vi "Process.vi"(8 "error in":errorcluster, 11 "SMO.Dictionary":refnum<class "SMO.Dictionary.lvclass">) -> (0 "error out":errorcluster, 3 "SMO.Dictionary out":refnum<class "SMO.Dictionary.lvclass">)   [LabVIEW 2013, in "SMO.Dictionary.lvlib" / "SMO.Dictionary.lvclass"]
doc: "---------------------------------------------------------------\nJKI State Machine Objects™\nhttp://jki.net/state-machine-objects/\nCopyright (C) 2005-2015, JKI <info@jki.net>\nALL RIGHTS RESERVED"
uses:
  SMO.Dictionary.lvclass
  <vilib>/JKI/JKI SMO/SMO/Typedefs/Parent Call--Enum.ctl
  <vilib>/JKI/JKI SMO/SMO/SMO.lvclass
  Typedefs/PrivateEvents--SMO.Dictionary.KeyValue-Pair.ctl
  Typedefs/PrivateEvents--SMO.Dictionary.GetMultipleValues.ctl
  Typedefs/PrivateEvents--SMO.Dictionary.KeyValue-Pair Array.ctl
  Typedefs/PrivateEvents--SMO.Dictionary.Get.ctl
  <vilib>/JKI/JKI SMO/SMO/SMO.lvclass/SMO.ctl
  <vilib>/JKI/JKI SMO/SMO/Private/ReftoDVR--SMO.vi
panel:
  # "For instructions on how to use the JKI State Machine Objects, examples and video tutorials, visit:\nhttp://jki.net/state-machine-objects/\n\nJKI State Machine Objects™\nhttp://jki.net/state-machine-objects/\nCopyright (C) 2005-2015, JKI <info@jki.net>\nALL RIGHTS RESERVED"
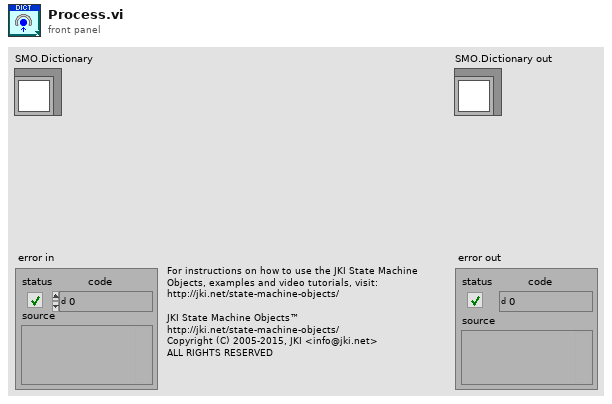
[diagram p1: front panel]
types:
  T1 = typedef "SMO.lvclass/Parent Call--Enum.ctl" = enum16{"Allows parent to run", "Does not request parent to run"}
  T2 = enum32{"invalid app kind", "Development System", "Run Time System", "Student Edition", "Embedded LabVIEW", "Evaluation", "Custom"}
  T3 = enum32{"Invalid", "Standard", "Closed", "Hidden", "Minimized", "Maximized"}
  T4 = enum32{"Bad", "Idle", "Run top level", "Running"}
  T5 = typedef "SMO.Dictionary.lvlib/SMO.Dictionary.lvclass/PrivateEvents--SMO.Dictionary.KeyValue-Pair.ctl" = cluster{"Key":string, "Value":variant}
  T6 = typedef "SMO.Dictionary.lvlib/SMO.Dictionary.lvclass/PrivateEvents--SMO.Dictionary.KeyValue-Pair Array.ctl" = cluster{"Keys":string[], "Values":variant[]}
  T7 = typedef "SMO.Dictionary.lvlib/SMO.Dictionary.lvclass/PrivateEvents--SMO.Dictionary.Get.ctl" = cluster{"Key":string, "response":refnum<notifier>}
  T8 = typedef "SMO.Dictionary.lvlib/SMO.Dictionary.lvclass/PrivateEvents--SMO.Dictionary.GetMultipleValues.ctl" = cluster{"Keys":string[], "response":refnum<notifier>}
  T9 = cluster{"Core":cluster{"Current VI Reference":refnum<vi>, "Close Panel on Exit?":bool, "error":errorcluster}, "Self Reference":refnum<class "SMO.Dictionary.lvclass">, "KeyValue Pair":T5, "Get":T7, "GetMultiple":T8}
  T10 = cluster{"Current VI Reference":refnum<vi>, "Close Panel on Exit?":bool, "error":errorcluster}
  T11 = typedef "SMO.lvclass/Protected Events.ctl" = cluster{"StopProcesses":refnum<user-event>, "AbortProcesses":refnum<user-event>, "Config Changed":refnum<user-event>, "Dependency":refnum<user-event>}
  T12 = typedef "SMO.Dictionary.lvlib/SMO.Dictionary.lvclass/PrivateEvents--Cluster.ctl" = cluster{"Update":refnum<user-event>, "Clear Dictionary":refnum<user-event>, "Delete":refnum<user-event>, "Get":refnum<user-event>, "GetMultiple":refnum<user-event>}
  T13 = typedef "SMO.Dictionary.lvlib/SMO.Dictionary.lvclass/PublicEvents--Cluster.ctl" = cluster{"Cleared":refnum<user-event>, "Deleted":refnum<user-event>, "Updated":refnum<user-event>}
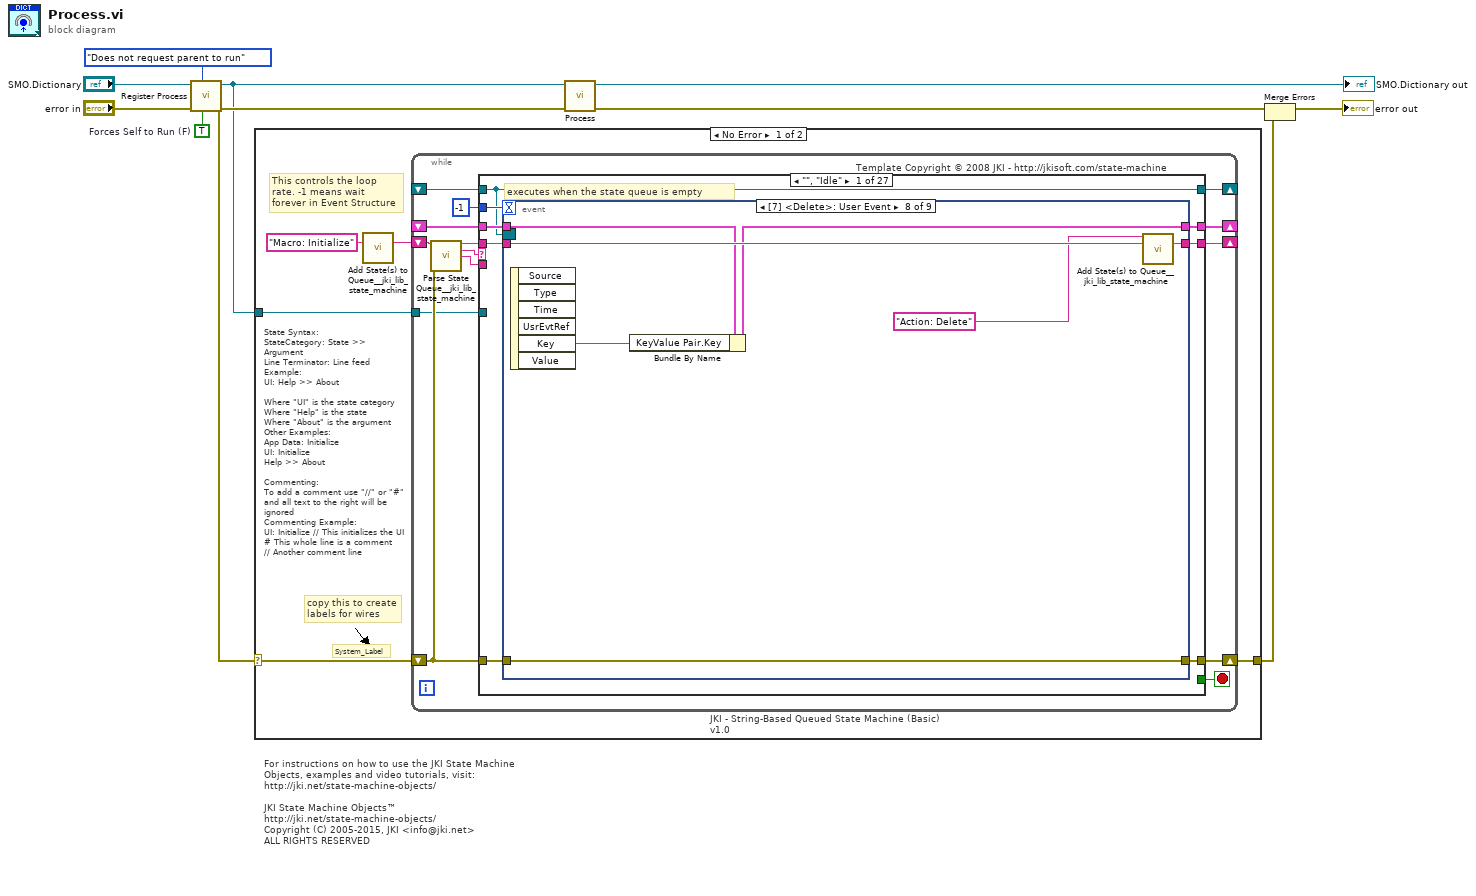
[diagram p0: block diagram]
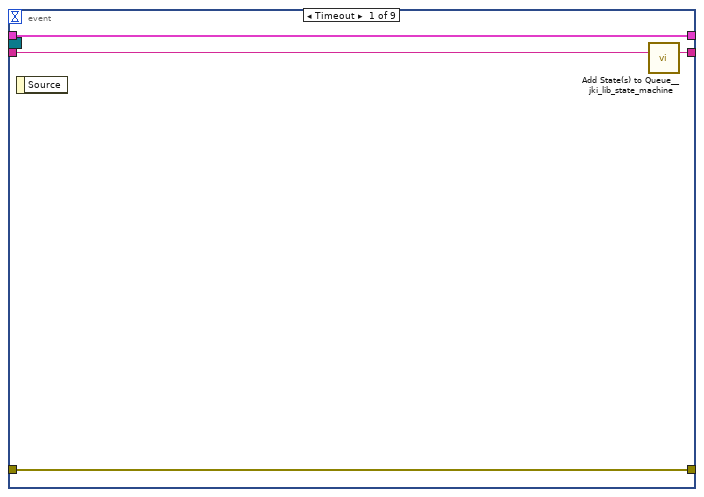
[diagram p2: hidden frame]
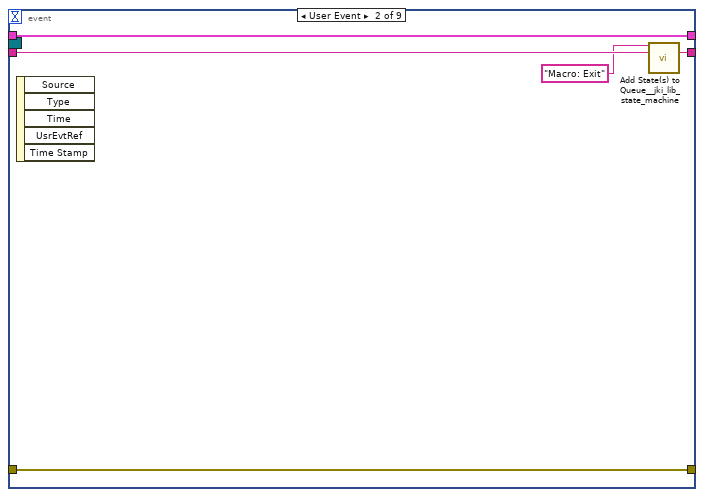
[diagram p3: hidden frame]
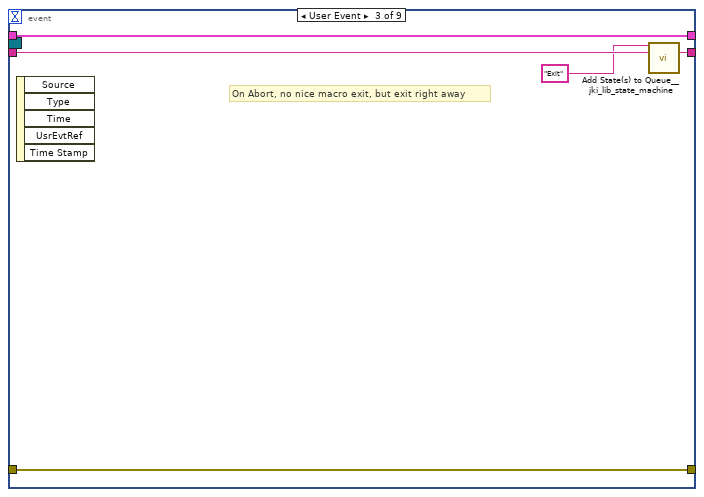
[diagram p4: hidden frame]
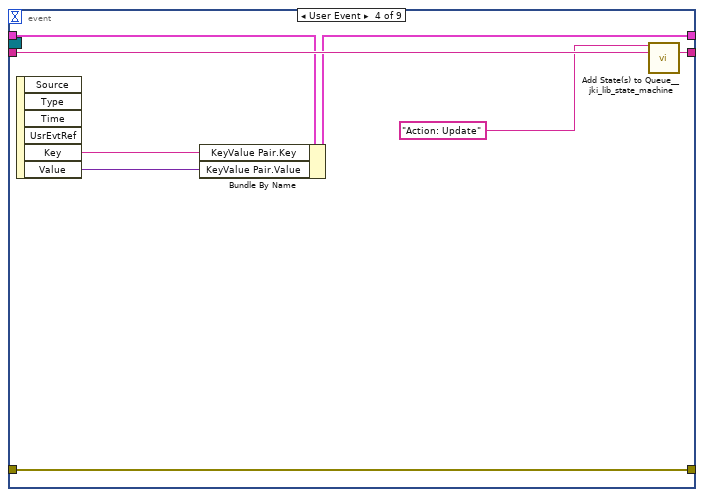
[diagram p5: hidden frame]
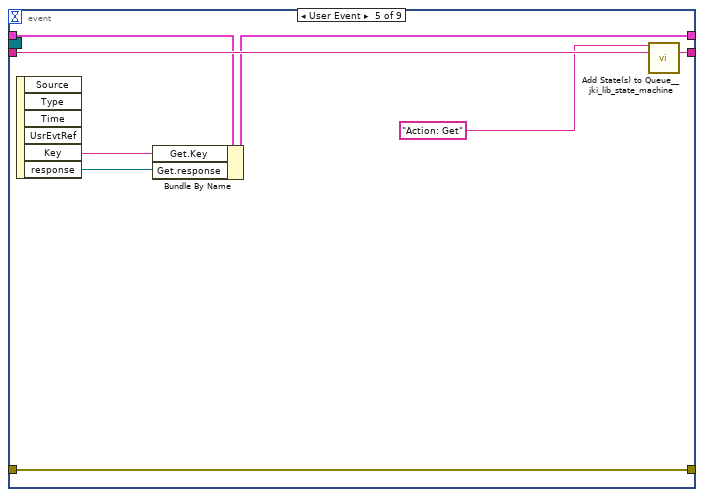
[diagram p6: hidden frame]
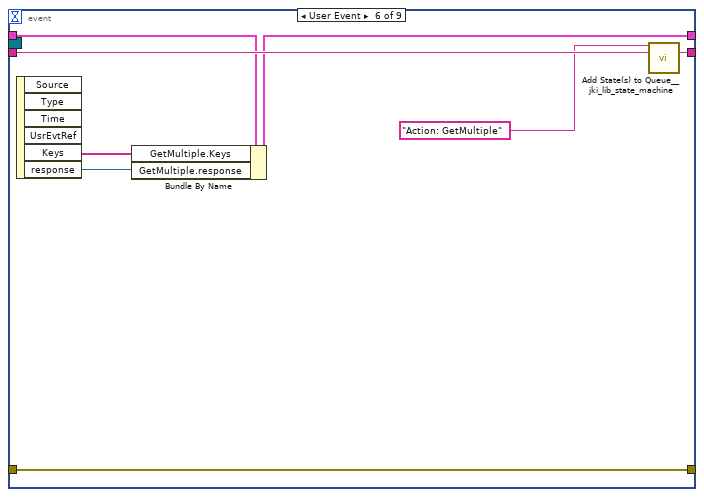
[diagram p7: hidden frame]
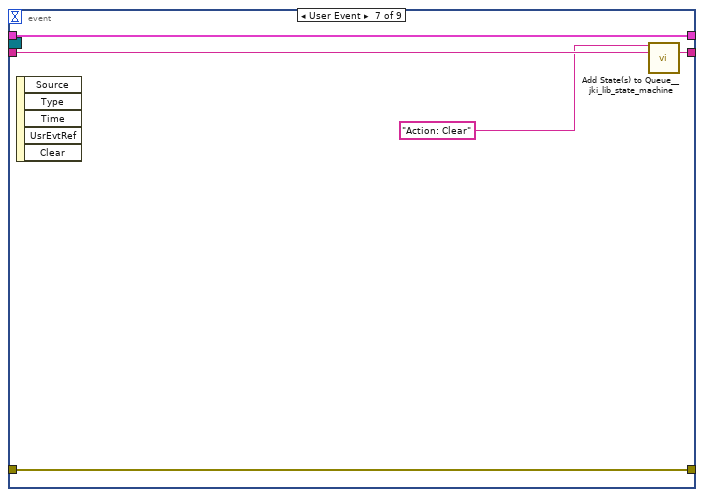
[diagram p8: hidden frame]
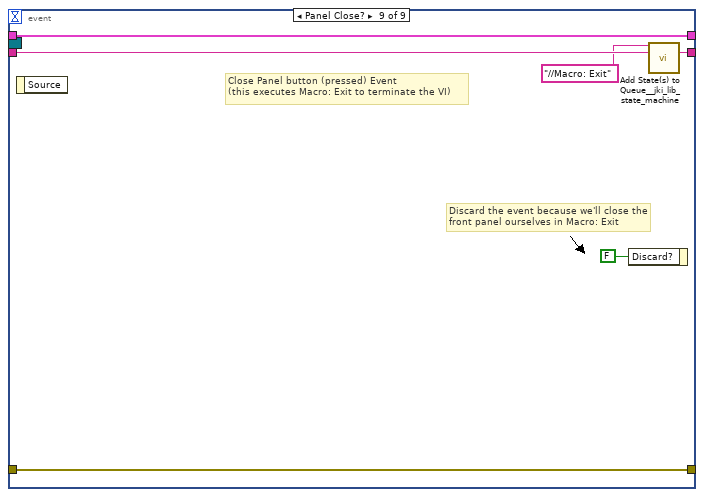
[diagram p9: hidden frame]
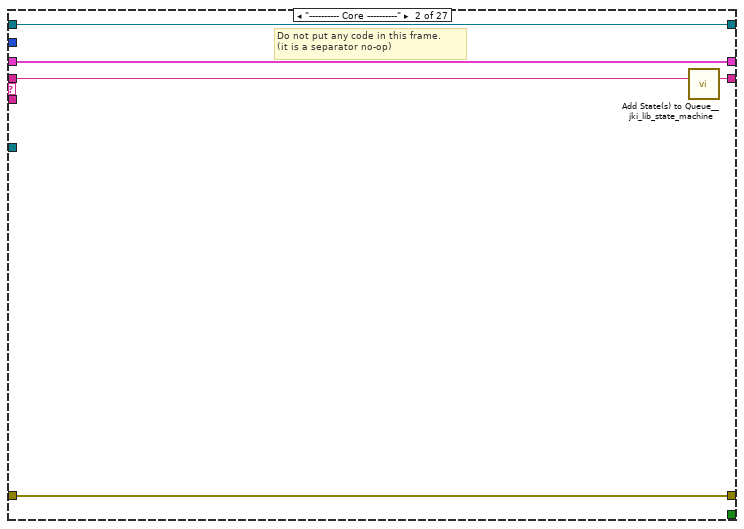
[diagram p10: hidden frame]
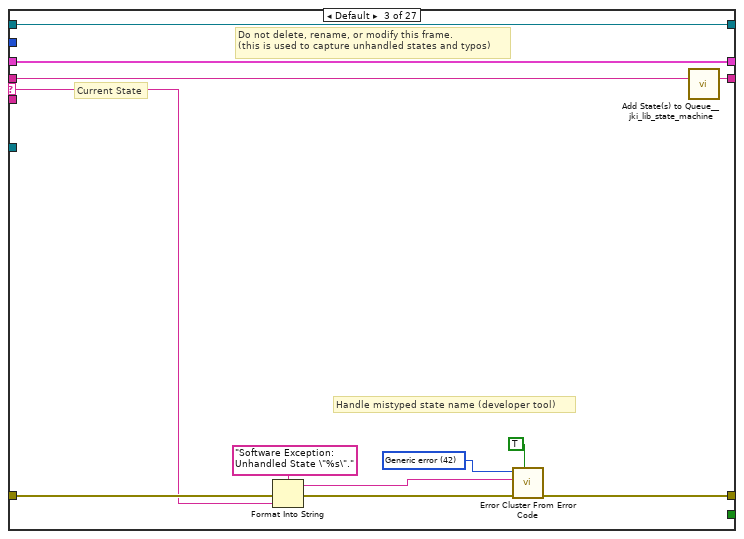
[diagram p11: hidden frame]
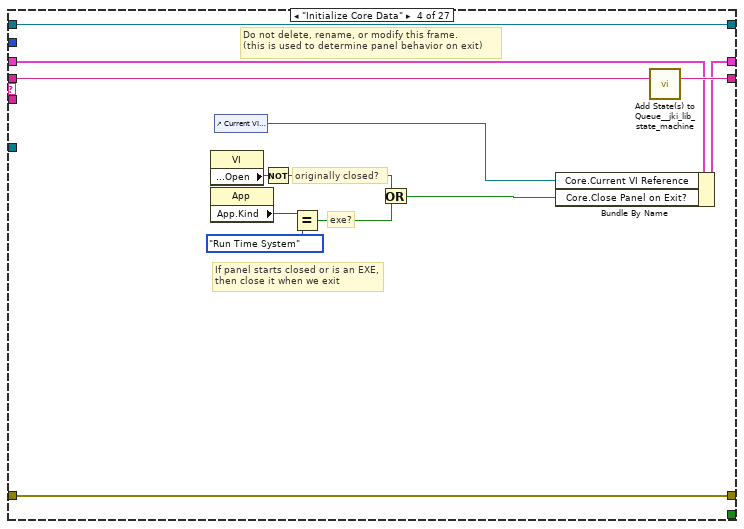
[diagram p12: hidden frame]
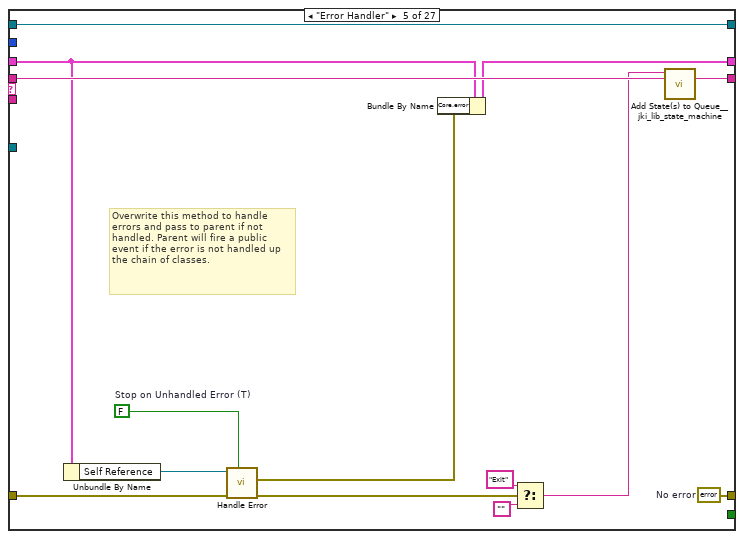
[diagram p13: hidden frame]
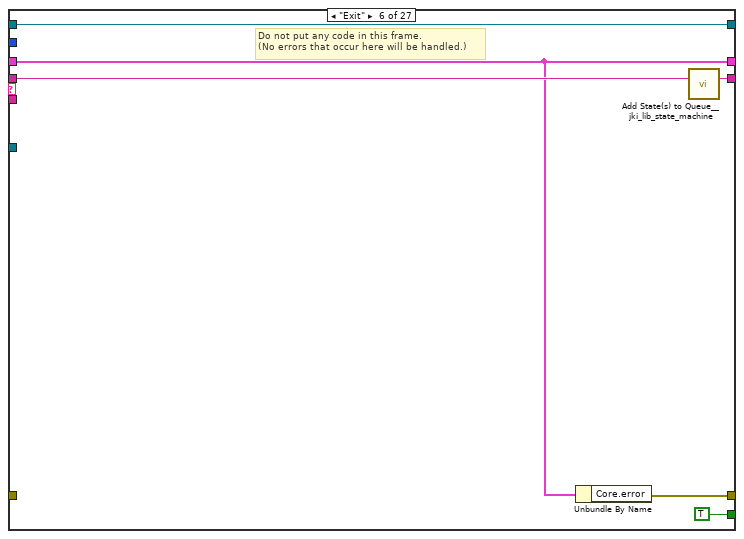
[diagram p14: hidden frame]
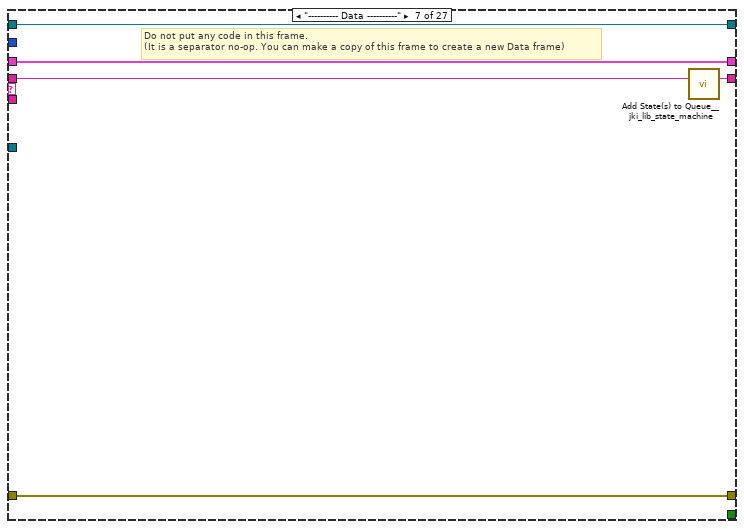
[diagram p15: hidden frame]
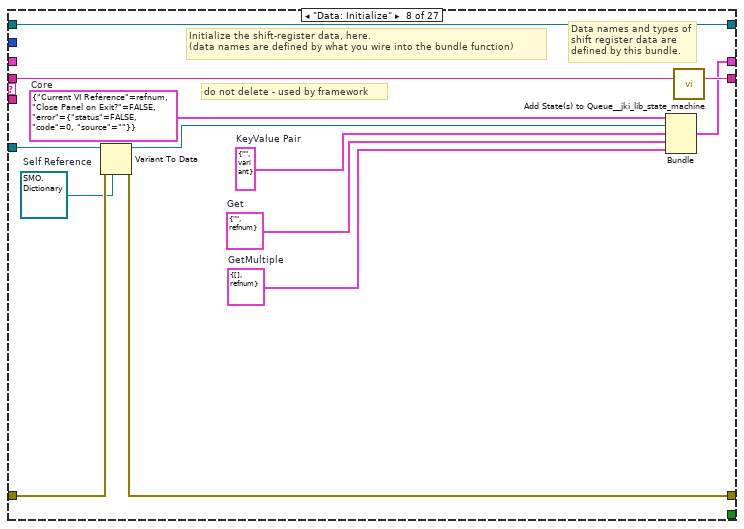
[diagram p16: hidden frame]
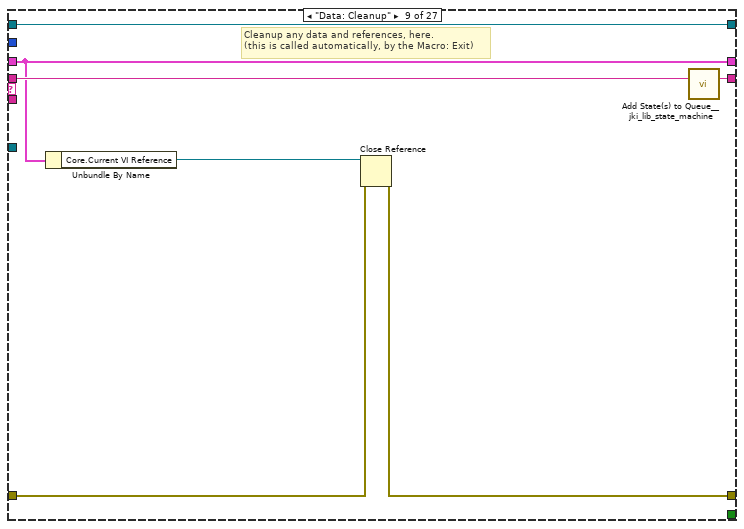
[diagram p17: hidden frame]
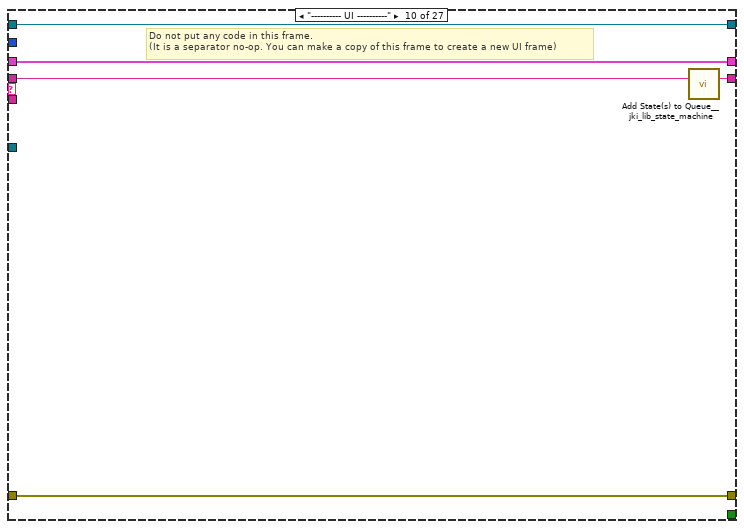
[diagram p18: hidden frame]
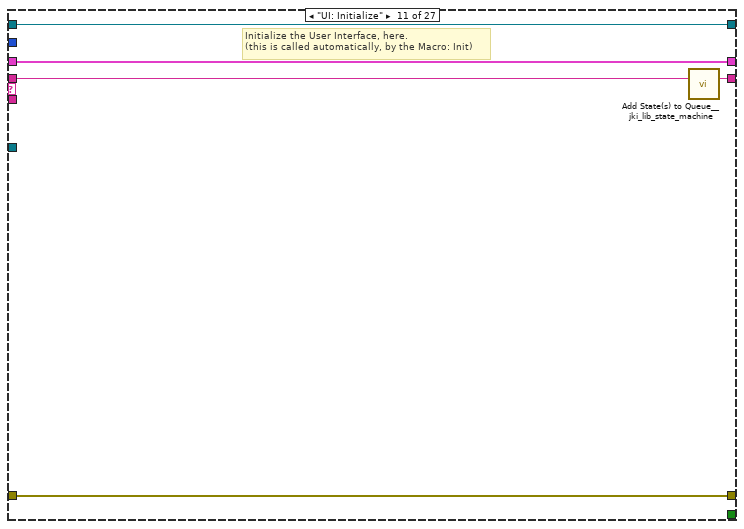
[diagram p19: hidden frame]
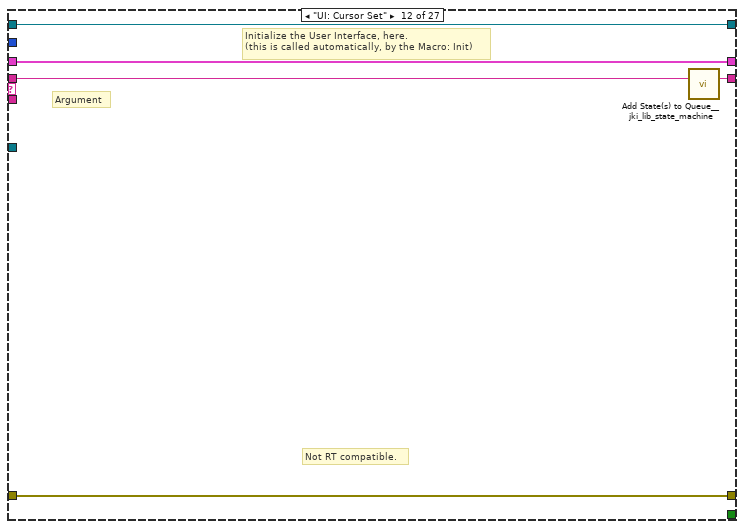
[diagram p20: hidden frame]
diagram:
  w1 = TRUE  # Forces Self to Run (F)
  # "For instructions on how to use the JKI State Machine Objects, examples and video tutorials, visit:\nhttp://jki.net/state-machine-objects/\n\nJKI State Machine Objects™\nhttp://jki.net/state-machine-objects/\nCopyright (C) 2005-2015, JKI <info@jki.net>\nALL RIGHTS RESERVED"
  n1 = call <vilib>:"Register Process.vi"("Forces Self to Run (F)"=w1, "Parent Call"=Parent_Call--Enum."Does not request parent to run", "error in (no error)"="error in", "SMO"="SMO.Dictionary") -> ("error out"=w7:errorcluster, "SMO out"=w6:refnum<class "SMO.Dictionary.lvclass">)  [unwired: 6 in]
  n2 = case shown="No Error" w7 {
    selector: w7 -> [w12 w372]
    tunnel: w6 -> [w13 _]
    tunnel: [w11 w372] -> w3
    frame No Error {
      # "State Syntax:\nStateCategory: State >> Argument\nLine Terminator: Line feed\nExample:\nUI: Help >> About\n\nWhere \"UI\" is the state category\nWhere \"Help\" is the state\nWhere \"About\" is the argument\nOther Examples:\nApp Data: Initialize\nUI: Initialize\nHelp >> About\n\nCommenting:\nTo add a comment use \"//\" or \"#\" and all text to the right will be ignored\nCommenting Example:\nUI: Initialize // This initializes the UI\n# This whole line is a comment\n// Another comment line"
      # "copy this to create labels for wires"
      # "This controls the loop rate. -1 means wait forever in Event Structure"
      # "System_Label"
      n3 = call <vilib>:"Add State(s) to Queue__jki_lib_state_machine.vi"("State(s) in (\"\")"="Macro: Initialize") -> ("States Out"=w15:string)  [unwired: 14 in]
      n4 = while "JKI - String-Based Queued State Machine (Basic) v1.0" {
        shift-right: [w22] -> _
        shift-left: _ -> [w21]
        shift-right: [w25] -> w11
        shift-left: w12 -> [w19]
        shift-right: [w24] -> _
        shift-left: w15 -> [w26]
        tunnel: w13 -> [w18]
        shift-right: [w17] -> _
        shift-left: _ -> [w16]
        stop <- w23 stop-if-true
        # "Template Copyright © 2008 JKI - http://jkisoft.com/state-machine"
        n5 = call <vilib>:"Parse State Queue__jki_lib_state_machine.vi"("State Queue"=w26, "Error In (no error)"=w19) -> ("Remaining States"=w28:string, "Current State"=w29:string, "Arguments"=w27:string)  [unwired: 11 in]
        n6 = case shown="\"\", \"Idle\"" w29 {
          selector: w29 -> [_ _ w100 _ _ _ _ _ _ _ _ _ _ _ _ _ _ _ _ _ _ _ _ _ _ _ _]
          tunnel: w28 -> [w37 w98 w104 w123 w137 w143 w148 w161 w168 w173 w178 w183 w191 w223 w237 w251 w256 w267 w272 w292 w298 w303 w314 w330 w346 w356 w371]
          tunnel: w27 -> [_ _ _ _ _ _ _ _ _ _ _ _ w185 _ _ _ _ _ _ _ _ _ _ _ _ _ _]
          tunnel: w21 -> [w35 w95 w102 w114 w131 w139 w145 _ w163 w170 w176 w181 w187 w220 w233 w242 w253 w264 w269 w290 w296 w301 w311 w327 w343 w353 w368]
          tunnel: [w34 w96 w106 w120 w132 w138 w146 w157 w164 w171 w175 w179 w188 w221 w235 w249 w254 w258 w270 w283 w294 w299 w304 w317 w341 w347 w358] -> w25
          tunnel: w19 -> [w33 w96 w105 w120 w133 _ w146 w158 w165 w171 w175 w179 w189 w221 w235 w249 w254 w259 w270 w287 w294 w299 w308 w315 w333 w349 w365]
          tunnel: [w36 w97 w103 w122 w136 w142 w147 w160 w167 w172 w177 w182 w190 w222 w236 w250 w255 w266 w271 w291 w297 w302 w313 w329 w345 w355 w370] -> w24
          tunnel: [_ _ _ _ _ TRUE _ _ _ _ _ _ _ _ _ _ _ _ _ _ _ _ _ _ _ _ _] -> w23
          tunnel: [w32 w95 w102 w121 w130 w139 w145 w159 w163 w170 w176 w181 w187 w220 w233 w242 w253 w264 w269 w290 w296 w301 w310 w326 w342 w352 w367] -> w22
          tunnel: -1 ("Timeout") -> [w31 _ _ _ _ _ _ _ _ _ _ _ _ _ _ _ _ _ _ _ _ _ _ _ _ _ _]
          tunnel: w18 -> [_ _ _ _ _ _ _ w155 _ _ _ _ _ _ _ _ _ _ _ _ _ _ _ _ _ _ _]
          tunnel: [w30 w94 w99 w111 w135 w140 w144 w153 w162 w169 w174 w180 w184 w219 w234 w243 w252 w265 w268 w273 w295 w300 w312 w328 w344 w354 w369] -> w17
          tunnel: w16 -> [w30 w94 w99 w111 w135 w140 w144 w153 w162 w169 w174 w180 w184 w219 w234 w243 w252 w265 w268 _ w295 w300 w312 w328 w344 w354 w369]
          frame "", "Idle" {
            # "executes when the state queue is empty"
            n7 = event shown="[7] <Delete>: User Event" {
              selector: w30 -> [_ _ _ _ _ _ _ _ _]
              dyn-events: _ -> [_ _ _ _ _ _ _ _ _]
              timeout: w31 -> [_ _ _ _ _ _ _ _ _]
              tunnel: w37 -> [w41 w46 w51 w59 w67 w75 w80 w87 w93]
              tunnel: [w40 w45 w50 w58 w66 w74 w79 w86 w92] -> w36
              tunnel: w35 -> [w39 w43 w48 w54 w62 w71 w76 w82 w90]
              tunnel: [w38 w44 w49 w57 w65 w73 w78 w85 w91] -> w34
              tunnel: w33 -> [w38 w44 w49 w57 w65 w73 w78 w85 w91]
              tunnel: [w39 w43 w48 w53 w61 w70 w76 w81 w90] -> w32
              event Timeout {
                n8 = event-data() -> ()  [unwired: 1 in, 1 out]
                n9 = call <vilib>:"Add State(s) to Queue__jki_lib_state_machine.vi"("State(s) in (\"\")"=w41) -> ("States Out"=w40:string)  [unwired: 14 in]
              }
              event User Event {
                n10 = event-data() -> ()  [unwired: 1 in, 5 out]
                n11 = call <vilib>:"Add State(s) to Queue__jki_lib_state_machine.vi"("State(s) in Front (\"\")"="Macro: Exit", "State(s) in (\"\")"=w46) -> ("States Out"=w45:string)  [unwired: 13 in]
              }
              event User Event {
                # "On Abort, no nice macro exit, but exit right away"
                n12 = event-data() -> ()  [unwired: 1 in, 5 out]
                n13 = call <vilib>:"Add State(s) to Queue__jki_lib_state_machine.vi"("State(s) in Front (\"\")"="Exit", "State(s) in (\"\")"=w51) -> ("States Out"=w50:string)  [unwired: 13 in]
              }
              event User Event {
                n14 = event-data() -> ("Key"=w56:string, "Value"=w55:variant)  [unwired: 1 in, 4 out]
                n15 = Bundle By Name(cluster=w54, "KeyValue Pair.Key"=w56, "KeyValue Pair.Value"=w55) -> (w53:T9)
                n16 = call <vilib>:"Add State(s) to Queue__jki_lib_state_machine.vi"("State(s) in Front (\"\")"="Action: Update", "State(s) in (\"\")"=w59) -> ("States Out"=w58:string)  [unwired: 13 in]
              }
              event User Event {
                n17 = event-data() -> ("Key"=w64:string, "response"=w63:refnum<notifier>)  [unwired: 1 in, 4 out]
                n18 = Bundle By Name(cluster=w62, "Get.Key"=w64, "Get.response"=w63) -> (w61:T9)
                n19 = call <vilib>:"Add State(s) to Queue__jki_lib_state_machine.vi"("State(s) in Front (\"\")"="Action: Get", "State(s) in (\"\")"=w67) -> ("States Out"=w66:string)  [unwired: 13 in]
              }
              event User Event {
                n20 = event-data() -> ("Keys"=w72:string[], "response"=w68:refnum<notifier>)  [unwired: 1 in, 4 out]
                n21 = Bundle By Name(cluster=w71, "GetMultiple.Keys"=w72, "GetMultiple.response"=w68) -> (w70:T9)
                n22 = call <vilib>:"Add State(s) to Queue__jki_lib_state_machine.vi"("State(s) in Front (\"\")"="Action: GetMultiple", "State(s) in (\"\")"=w75) -> ("States Out"=w74:string)  [unwired: 13 in]
              }
              event User Event {
                n23 = event-data() -> ()  [unwired: 1 in, 5 out]
                n24 = call <vilib>:"Add State(s) to Queue__jki_lib_state_machine.vi"("State(s) in Front (\"\")"="Action: Clear", "State(s) in (\"\")"=w80) -> ("States Out"=w79:string)  [unwired: 13 in]
              }
              event User Event {
                n25 = event-data() -> ("Key"=w83:string)  [unwired: 1 in, 5 out]
                n26 = Bundle By Name(cluster=w82, "KeyValue Pair.Key"=w83) -> (w81:T9)
                n27 = call <vilib>:"Add State(s) to Queue__jki_lib_state_machine.vi"("State(s) in Front (\"\")"="Action: Delete", "State(s) in (\"\")"=w87) -> ("States Out"=w86:string)  [unwired: 13 in]
              }
              event Panel Close? {
                # "Discard the event because we'll close the front panel ourselves in Macro: Exit"
                # "Close Panel button (pressed) Event\n(this executes Macro: Exit to terminate the VI)"
                n28 = event-data() -> ()  [unwired: 1 in, 1 out]
                n29 = event-data("Discard?"=FALSE) -> ()  [unwired: 1 in, 1 out]
                n30 = call <vilib>:"Add State(s) to Queue__jki_lib_state_machine.vi"("State(s) in Front (\"\")"="//Macro: Exit", "State(s) in (\"\")"=w93) -> ("States Out"=w92:string)  [unwired: 13 in]
              }
            }
          }
          frame "---------- Core ----------" {
            # "Do not put any code in this frame.\n(it is a separator no-op)"
            n31 = call <vilib>:"Add State(s) to Queue__jki_lib_state_machine.vi"("State(s) in (\"\")"=w98) -> ("States Out"=w97:string)  [unwired: 14 in]
          }
          frame Default {
            w109 = 42 items=["No error", "Argument error", "Memory is full", "Out of zone", "End of file", "File already open", "Generic file I/O error", "File not found", "File permission error", "Disk is full", "Duplicate path", "Too many files open", "System feature not enabled", "Resource file not found", "Cannot add resource", "Resource not found", "Image not found", "Image memory error", "Pen does not exist", "Config type invalid", "Config token not found", "Config parse error", "Config memory error", "Bad external code format", "Bad external code offset", "External code not present", "Null window", "Destroy window error", "Null menu", "Print aborted", "Bad print record", "Print driver error", "Windows error during printing", "Memory error during printing", "Print dialog error", "Generic print error", "Invalid device refnum", "Device not found", "Device parameter error", "Device unit error", "Cannot open device", "Device call aborted", "Generic error", "Cancelled by user", "Object ID too low", "Object ID too high", "Object not in heap", "Unknown heap", "Unknown object (invalid DefProc)", "Unknown object (DefProc not in table)", "Message out of range", "Invalid (null) method", "Unknown message", "Manager call not supported", "Bad address", "Network operation in progress", "Network operation timed out", "Connection is busy", "Network attribute not supported", "Network error", "Address in use", "System out of memory", "Connection aborted", "Connection refused", "Not connected", "Already connected", "Connection closed", "Initialization error (interapplication manager)", "Bad occurrence", "Wait on unbound occurrence handler", "Occurrence queue overflow", "Datalog type conflict", "Unused", "Unrecognized type (interapplication manager)", "Memory corrupt", "Failed to make temporary DLL", "Old CIN version", "Drag socket not found", "Failed to load drop-object", "Failed to register OLE object", "Failed to release OLE object", "Format specifier type mismatch", "Unknown format specifier", "Too few format specifiers", "Too many format specifiers", "Scan failed", "Newer CIN version", "Error converting to variant", "Runtime menu error", "Password tampered", "Variant attribute not found", "Incompatible variant data type", "Event data is not available", "Event Store is not present", "Occurrence is not found", "Event Queue is not created", "Event info is not available", "Refnum passed is NULL", "Error retrieving Class GUID", "Error retrieving CoClass GUID", "Error retrieving TypeLib GUID.", "Bad built application magic bytes.", "Specific driver is different from the specific driver associated with the Logical Name.", "There is no session opened to the class driver.", "Max Error", "MAX - Error with config objects", "MAX - Error loading configuration", "MAX - Group not supported"]
            # "Current State"
            # "Do not delete, rename, or modify this frame.\n(this is used to capture unhandled states and typos)"
            # "Handle mistyped state name (developer tool)"
            n32 = Format Into String(format string="Software Exception: Unhandled State \"%s\"." ("message"), error in=w105, w100) -> (resulting string=w108:string, error out=w107:errorcluster)  [unwired: 1 in]
            n33 = call <vilib>:"Error Cluster From Error Code.vi"("show call chain? (False)"=TRUE, "error in (no error)"=w107, "error message (\"\")"=w108, "error code (0)"=w109) -> ("error out"=w106:errorcluster)  [unwired: 5 in]
            n34 = call <vilib>:"Add State(s) to Queue__jki_lib_state_machine.vi"("State(s) in (\"\")"=w104) -> ("States Out"=w103:string)  [unwired: 14 in]
          }
          frame "Initialize Core Data" {
            # "Do not delete, rename, or modify this frame.\n(this is used to determine panel behavior on exit)"
            # "originally closed?"
            # "exe?"
            # "If panel starts closed or is an EXE, then close it when we exit"
            n35 = property class="VI"() -> ("Front Panel.Open"=w119:bool)  [unwired: 2 in, 2 out]
            n36 = property class="App"() -> ("App.Kind"=w118:T2)  [unwired: 2 in, 2 out]
            n37 = control-ref of="Current VI Reference"() -> (w112:refnum<vi>)
            n38 = Not(x=w119) -> (.not. x?=w116:bool)
            n39 = Equal?(x=w118, y=T2."Run Time System" ("Application:Kind")) -> (x = y?=w115:bool)
            n40 = Or(x=w116, y=w115) -> (x .or. y?=w113:bool)
            n41 = Bundle By Name(cluster=w114, "Core.Current VI Reference"=w112, "Core.Close Panel on Exit?"=w113) -> (w121:T9)
            n42 = call <vilib>:"Add State(s) to Queue__jki_lib_state_machine.vi"("State(s) in (\"\")"=w123) -> ("States Out"=w122:string)  [unwired: 14 in]
          }
          frame "Error Handler" {
            w124 = FALSE  # Stop on Unhandled Error (T)
            w132 = errorcluster {"status"=FALSE, "code"=0, "source"=""}  # No error
            # "Overwrite this method to handle errors and pass to parent if not handled. Parent will fire a public event if the error is not handled up the chain of classes."
            n43 = Unbundle By Name(w131) -> ("Self Reference"=w134:refnum<class "SMO.Dictionary.lvclass">)
            n44 = call-dynamic "Handle Error.vi"("Stop on Unhandled Error (T)"=w124, "error in"=w133, "SMO.Dictionary"=w134) -> ("handling error"=w125:errorcluster, "Unhandled error"=w128:errorcluster)  [unwired: 6 in, 1 out]
            n45 = Bundle By Name(cluster=w131, "Core.error"=w128) -> (w130:T9)
            n46 = Select(t="Exit", s=w125, f="") -> (s? t:f=w129:string)
            n47 = call <vilib>:"Add State(s) to Queue__jki_lib_state_machine.vi"("State(s) in Front (\"\")"=w129, "State(s) in (\"\")"=w137) -> ("States Out"=w136:string)  [unwired: 13 in]
          }
          frame "Exit" {
            # "Do not put any code in this frame.\n(No errors that occur here will be handled.)"
            n48 = Unbundle By Name(w139) -> ("Core.error"=w138:errorcluster)
            n49 = call <vilib>:"Add State(s) to Queue__jki_lib_state_machine.vi"("State(s) in (\"\")"=w143) -> ("States Out"=w142:string)  [unwired: 14 in]
          }
          frame "---------- Data ----------" {
            # "Do not put any code in this frame.\n(It is a separator no-op. You can make a copy of this frame to create a new Data frame)"
            n50 = call <vilib>:"Add State(s) to Queue__jki_lib_state_machine.vi"("State(s) in (\"\")"=w148) -> ("States Out"=w147:string)  [unwired: 14 in]
          }
          frame "Data: Initialize" {
            w149 = T7 {"Key"="", "response"=refnum}  # Get
            w150 = T8 {"Keys"=[], "response"=refnum}  # GetMultiple
            w151 = T5 {"Key"="", "Value"=variant}  # KeyValue Pair
            w152 = T10 {"Current VI Reference"=refnum, "Close Panel on Exit?"=FALSE, "error"={"status"=FALSE, "code"=0, "source"=""}}  # Core
            w156 = refnum<class "SMO.Dictionary.lvclass"> refnum  # Self Reference
            # "do not delete - used by framework"
            # "Data names and types of shift register data are defined by this bundle."
            # "Initialize the shift-register data, here.\n(data names are defined by what you wire into the bundle function)"
            n51 = Variant To Data(error in=w158, type=w156, Variant=w155) -> (data=w154:refnum<class "SMO.Dictionary.lvclass">, error out=w157:errorcluster)
            n52 = Bundle("Core"=w152, "Self Reference"=w154, "KeyValue Pair"=w151, "Get"=w149, "GetMultiple"=w150) -> (w159:T9)  [unwired: 1 in]
            n53 = call <vilib>:"Add State(s) to Queue__jki_lib_state_machine.vi"("State(s) in (\"\")"=w161) -> ("States Out"=w160:string)  [unwired: 14 in]
          }
          frame "Data: Cleanup" {
            # "Cleanup any data and references, here.\n(this is called automatically, by the Macro: Exit)"
            n54 = Unbundle By Name(w163) -> ("Core.Current VI Reference"=w166:refnum<vi>)
            n55 = Close Reference(reference=w166, error in (no error)=w165) -> (error out=w164:errorcluster)
            n56 = call <vilib>:"Add State(s) to Queue__jki_lib_state_machine.vi"("State(s) in (\"\")"=w168) -> ("States Out"=w167:string)  [unwired: 14 in]
          }
          frame "---------- UI ----------" {
            # "Do not put any code in this frame.\n(It is a separator no-op. You can make a copy of this frame to create a new UI frame)"
            n57 = call <vilib>:"Add State(s) to Queue__jki_lib_state_machine.vi"("State(s) in (\"\")"=w173) -> ("States Out"=w172:string)  [unwired: 14 in]
          }
          frame "UI: Initialize" {
            # "Initialize the User Interface, here.\n(this is called automatically, by the Macro: Init)"
            n58 = call <vilib>:"Add State(s) to Queue__jki_lib_state_machine.vi"("State(s) in (\"\")"=w178) -> ("States Out"=w177:string)  [unwired: 14 in]
          }
          frame "UI: Cursor Set" {
            # "Not RT compatible."
            # "Argument"
            # "Initialize the User Interface, here.\n(this is called automatically, by the Macro: Init)"
            n59 = call <vilib>:"Add State(s) to Queue__jki_lib_state_machine.vi"("State(s) in (\"\")"=w183) -> ("States Out"=w182:string)  [unwired: 14 in]
          }
          frame "UI: Front Panel State" {
            # "Argument"
            # "Set Front Panel Open or Closed\n(Usage: \"UI: Front Panel State >> Open|Close\")"
            n60 = Unbundle By Name(w187) -> ("Core.Current VI Reference"=w186:refnum<vi>)
            n61 = disable-structure shown="Default" {
              disable-tunnel: w189 -> [w195 w218]
              disable-tunnel: [w194 w218] -> w188
              disable-tunnel: w186 -> [w193 _]
              disable-tunnel: w185 -> [w192 _]
              frame condition #0 (active) {
                n62 = case shown="\"Close\"" w192 {
                  tunnel: w195 -> [w199 w212]
                  tunnel: [w201 w213] -> w194
                  tunnel: w193 -> [w200 w210]
                  frame "Open", Default {
                    n63 = property class="VI"(reference=w200, error in=w199) -> (reference out=w197:refnum<vi>, error out=w198:errorcluster, "FP.State"=w196:T3)
                    n64 = case shown="\"Closed\"" w196 {
                      tunnel: [w204 w207] -> w201
                      tunnel: w198 -> [w203 w207]
                      tunnel: w197 -> [w202 _]
                      frame "Closed" {
                        n65 = invoke class="VI" method="FP.Open"(reference=w202, error in=w203, "Activate"=TRUE, "State"=T3."Standard") -> (error out=w204:errorcluster)  [unwired: 1 in, 4 out]
                      }
                      frame Default {
                      }
                    }
                  }
                  frame "Close" {
                    n66 = property class="VI"(reference=w210, error in=w212) -> (reference out=w209:refnum<vi>, error out=w211:errorcluster, "FP.State"=w208:T3)
                    n67 = case shown="Default" w208 {
                      tunnel: [w214 w217] -> w213
                      tunnel: w211 -> [w214 w216]
                      tunnel: w209 -> [_ w215]
                      frame "Invalid", "Closed" {
                      }
                      frame Default {
                        n68 = invoke class="VI" method="FP.Close"(reference=w215, error in=w216) -> (error out=w217:errorcluster)  [unwired: 1 in, 2 out]
                      }
                    }
                  }
                }
              }
              frame condition #1 {
              }
            }
            n69 = call <vilib>:"Add State(s) to Queue__jki_lib_state_machine.vi"("State(s) in (\"\")"=w191) -> ("States Out"=w190:string)  [unwired: 14 in]
          }
          frame "---------- Macro ----------" {
            # "Do not put any code in this frame.\n(It is a separator no-op. You can make a copy of this frame to create a new Macro frame)"
            n70 = call <vilib>:"Add State(s) to Queue__jki_lib_state_machine.vi"("State(s) in (\"\")"=w223) -> ("States Out"=w222:string)  [unwired: 14 in]
          }
          frame "Macro: Initialize" {
            w228 = "//UI: Initialize\n//UI: Front Panel State >> Open"  # //UI: Initialize //UI: Front Panel State >> Open
            w224 = "Process: Sync"
            # "Initialization Macro\n(This is called once, when the VI starts)"
            n71 = control-ref of="This VI"() -> (w226:refnum<vi>)
            n72 = property class="VI"(reference=w226) -> ("Exec.State"=w225:T4)  [unwired: 1 in, 2 out]
            n73 = Equal?(x=w225, y=T4."Run top level") -> (x = y?=w231:bool)
            n74 = Select(t=w224, s=w231, f="") -> ()  [unwired: 1 out]
            n75 = call <vilib>:"Add State(s) to Queue__jki_lib_state_machine.vi"("State(s) in Front (\"\")"="Data: Initialize\nInitialize Core Data\nEvents: Register", "State(s) in (\"\")"=w224, "State(s) at Back (\"\")"=w228) -> ("States Out"=w227:string)  [unwired: 12 in]
            n76 = call <vilib>:"Add State(s) to Queue__jki_lib_state_machine.vi"("State(s) in Front (\"\")"=w227, "State(s) in (\"\")"=w237) -> ("States Out"=w236:string)  [unwired: 13 in]
          }
          frame "Macro: Exit" {
            # "Exit Macro\n(This is called once, when the VI exits)"
            n77 = Unbundle By Name(w242) -> ("Core.Close Panel on Exit?"=w248:bool)
            n78 = Select(t="UI: Front Panel State >> Close", s=w248, f="") -> (s? t:f=w245:string)
            n79 = call <vilib>:"Add State(s) to Queue__jki_lib_state_machine.vi"("State(s) in Front (\"\")"="Data: Cleanup\nEvents: Unregister", "State(s) in (\"\")"="Process: Sync", "State(s) at Back (\"\")"="Exit") -> ("States Out"=w239:string)  [unwired: 12 in]
            n80 = call <vilib>:"Add State(s) to Queue__jki_lib_state_machine.vi"("State(s) in (\"\")"=w245, "State(s) at Back (\"\")"=w239) -> ("States Out"=w244:string)  [unwired: 13 in]
            n81 = call <vilib>:"Add State(s) to Queue__jki_lib_state_machine.vi"("State(s) in Front (\"\")"=w244, "State(s) in (\"\")"=w251) -> ("States Out"=w250:string)  [unwired: 13 in]
          }
          frame "---------- Process ----------" {
            # "Template Separator\n(You can make a copy of, or modify, this frame)"
            n82 = call <vilib>:"Add State(s) to Queue__jki_lib_state_machine.vi"("State(s) in (\"\")"=w256) -> ("States Out"=w255:string)  [unwired: 14 in]
          }
          frame "Process: Sync" {
            n83 = Unbundle By Name(w264) -> ("Self Reference"=w260:refnum<class "SMO.Dictionary.lvclass">)
            n84 = call <vilib>:"WaitOnProcessSync.vi"("error in (no error)"=w259, "SMO"=w260) -> ("error out"=w258:errorcluster, "Don't run?"=w263:bool)  [unwired: 7 in, 1 out]
            n85 = Select(t="Data: Cleanup\nEvents: Unregister\nExit", s=w263, f="") -> (s? t:f=w257:string)
            n86 = call <vilib>:"Add State(s) to Queue__jki_lib_state_machine.vi"("State(s) in Front (\"\")"=w257, "State(s) in (\"\")"=w267) -> ("States Out"=w266:string)  [unwired: 13 in]
          }
          frame "---------- Events ----------" {
            # "Template Separator\n(You can make a copy of, or modify, this frame)"
            n87 = call <vilib>:"Add State(s) to Queue__jki_lib_state_machine.vi"("State(s) in (\"\")"=w272) -> ("States Out"=w271:string)  [unwired: 14 in]
          }
          frame "Events: Register" {
            # "Expand to add\nmore events"
            n88 = Unbundle By Name(w290) -> ("Self Reference"=w289:refnum<class "SMO.Dictionary.lvclass">)
            n89 = call <vilib>:"GetProtectedEvents.vi"("SMO"=w289) -> ("error out"=w285:errorcluster, "SMO Protected Events"=w282:T11, "SMO out"=w288:refnum<class "SMO.Dictionary.lvclass">)  [unwired: 8 in]
            n90 = call "SMO.Dictionary.GetPrivateEvents.vi"("SMO.Dictionary"=w288) -> ("error out"=w286:errorcluster, "Private Events"=w280:T12)  [unwired: 8 in, 1 out]
            n91 = Unbundle By Name(w282) -> ("StopProcesses"=w281:refnum<user-event>, "AbortProcesses"=w279:refnum<user-event>)
            n92 = Unbundle By Name(w280) -> ("Update"=w278:refnum<user-event>, "Get"=w277:refnum<user-event>, "GetMultiple"=w276:refnum<user-event>, "Clear Dictionary"=w275:refnum<user-event>, "Delete"=w274:refnum<user-event>)
            n93 = register-events(w281, w279, w278, w277, w276, w275, w274) -> (reference out=w273:refnum<event-registration>, error out=w284:errorcluster)  [unwired: 2 in]
            n94 = Merge Errors(w287, w284, w286, w285) -> (w283:errorcluster)
            n95 = call <vilib>:"Add State(s) to Queue__jki_lib_state_machine.vi"("State(s) in (\"\")"=w292) -> ("States Out"=w291:string)  [unwired: 14 in]
          }
          frame "Events: Unregister" {
            n96 = Unregister For Events(event registration refnum=w295, error in=w294) -> (error out=w293:errorcluster)
            n97 = call <vilib>:"Clear Errors.vi"("error in (no error)"=w293) -> ()  [unwired: 6 in, 1 out]
            n98 = call <vilib>:"Add State(s) to Queue__jki_lib_state_machine.vi"("State(s) in (\"\")"=w298) -> ("States Out"=w297:string)  [unwired: 14 in]
          }
          frame "---------- Action ----------" {
            n99 = call <vilib>:"Add State(s) to Queue__jki_lib_state_machine.vi"("State(s) in (\"\")"=w303) -> ("States Out"=w302:string)  [unwired: 14 in]
          }
          frame "Action: Update" {
            n100 = Unbundle By Name(w311) -> ("Self Reference"=w309:refnum<class "SMO.Dictionary.lvclass">, "KeyValue Pair.Key"=w307:string, "KeyValue Pair.Value"=w306:variant)  [unwired: 1 out]
            n101 = call-dynamic "Update Dictionary.vi"("error in (no error)"=w308, "Variant"=w306, "Key"=w307, "SMO.Dictionary in"=w309) -> ("error out"=w304:errorcluster, "SMO.Dictionary out"=w305:refnum<class "SMO.Dictionary.lvclass">)  [unwired: 6 in]
            n102 = Bundle By Name(cluster=w311, "Self Reference"=w305) -> (w310:T9)
            n103 = call <vilib>:"Add State(s) to Queue__jki_lib_state_machine.vi"("State(s) in (\"\")"=w314) -> ("States Out"=w313:string)  [unwired: 14 in]
          }
          frame "Action: Get" {
            n104 = Unbundle By Name(w327) -> ("Self Reference"=w325:refnum<class "SMO.Dictionary.lvclass">, "Get.Key"=w323:string, "Get.response"=w316:refnum<notifier>)
            n105 = call-dynamic "Get Element.vi"("error in (no error)"=w315, "Key"=w323, "SMO.Dictionary in"=w325) -> ("error out"=w318:errorcluster, "Value"=w320:variant, "Key dup"=w321:string, "SMO.Dictionary out"=w324:refnum<class "SMO.Dictionary.lvclass">)  [unwired: 5 in]
            n106 = Bundle By Name(cluster=T5 {"Key"="", "Value"=variant} ("Update"), "Key"=w321, "Value"=w320) -> (w319:T5)
            n107 = Send Notification(notification=w319, notifier=w316, error in (no error)=w318) -> (error out=w317:errorcluster)  [unwired: 1 out]
            n108 = Bundle By Name(cluster=w327, "Self Reference"=w324) -> (w326:T9)
            n109 = call <vilib>:"Add State(s) to Queue__jki_lib_state_machine.vi"("State(s) in (\"\")"=w330) -> ("States Out"=w329:string)  [unwired: 14 in]
          }
          frame "Action: GetMultiple" {
            n110 = Unbundle By Name(w343) -> ("Self Reference"=w340:refnum<class "SMO.Dictionary.lvclass">, "GetMultiple.Keys"=w334:string[], "GetMultiple.response"=w335:refnum<notifier>)
            n111 = call-dynamic "Get Elements.vi"("error in (no error)"=w333, "Keys (empty: All)"=w334, "SMO.Dictionary in"=w340) -> ("error out"=w332:errorcluster, "Values"=w338:variant[], "Keys out"=w339:string[], "SMO.Dictionary out"=w331:refnum<class "SMO.Dictionary.lvclass">)  [unwired: 5 in]
            n112 = Bundle By Name(cluster=T6 {"Keys"=[], "Values"=[]} ("KeyValue Pairs"), "Keys"=w339, "Values"=w338) -> (w336:T6)
            n113 = Bundle By Name(cluster=w343, "Self Reference"=w331) -> (w342:T9)
            n114 = Send Notification(notification=w336, notifier=w335, error in (no error)=w332) -> (error out=w341:errorcluster)  [unwired: 1 out]
            n115 = call <vilib>:"Add State(s) to Queue__jki_lib_state_machine.vi"("State(s) in (\"\")"=w346) -> ("States Out"=w345:string)  [unwired: 14 in]
          }
          frame "Action: Delete" {
            n116 = Unbundle By Name(w353) -> ("Self Reference"=w350:refnum<class "SMO.Dictionary.lvclass">, "KeyValue Pair.Key"=w351:string)
            n117 = call-dynamic "Delete Element.vi"("error in (no error)"=w349, "Key"=w351, "SMO.Dictionary in"=w350) -> ("error out"=w347:errorcluster, "SMO.Dictionary out"=w348:refnum<class "SMO.Dictionary.lvclass">)  [unwired: 6 in, 1 out]
            n118 = Bundle By Name(cluster=w353, "Self Reference"=w348) -> (w352:T9)
            n119 = call <vilib>:"Add State(s) to Queue__jki_lib_state_machine.vi"("State(s) in (\"\")"=w356) -> ("States Out"=w355:string)  [unwired: 14 in]
          }
          frame "Action: Clear" {
            n120 = Unbundle By Name(w368) -> ("Self Reference"=w366:refnum<class "SMO.Dictionary.lvclass">)
            n121 = call-dynamic "Clear Dictionary.vi"("error in (no error)"=w365, "SMO.Dictionary in"=w366) -> ("error out"=w362:errorcluster, "SMO.Dictionary out"=w364:refnum<class "SMO.Dictionary.lvclass">)  [unwired: 8 in]
            n122 = call "SMO.Dictionary.GetPublicEvents.vi"("error in (no error)"=w362, "SMO.Dictionary in"=w364) -> ("error out"=w359:errorcluster, "Public Events"=w361:T13, "SMO.Dictionary out"=w363:refnum<class "SMO.Dictionary.lvclass">)  [unwired: 7 in]
            n123 = Unbundle By Name(w361) -> ("Cleared"=w360:refnum<user-event>)
            n124 = Generate User Event(user event=w360, event data cluster=TRUE ("event data"), error in=w359) -> (error out=w358:errorcluster)  [unwired: 1 in, 1 out]
            n125 = Bundle By Name(cluster=w368, "Self Reference"=w363) -> (w367:T9)
            n126 = call <vilib>:"Add State(s) to Queue__jki_lib_state_machine.vi"("State(s) in (\"\")"=w371) -> ("States Out"=w370:string)  [unwired: 14 in]
          }
        }
      }
    }
    frame Error {
    }
  }
  n127 = call-parent "Process.vi"("error in"=w7, "SMO"=w6) -> ("error out"=w4:errorcluster, "SMO out"=→"SMO.Dictionary out":refnum<class "SMO.Dictionary.lvclass">)  [unwired: 8 in]
  n128 = Merge Errors(w4, w3) -> (→"error out":errorcluster)
